vi "subMFD_Design & Analysis.vi"() -> ()   [LabVIEW 2023]
uses:
  <vilib>/Utility/error.llb/ErrWarn.ctl
  <vilib>/addons/Digital Filter Design/_Objects.llb/DFD Filter Ripple Specification (Design).ctl
  <vilib>/addons/Digital Filter Design/_Objects.llb/DFD Multirate Filter Obj.ctl
  <vilib>/addons/Digital Filter Design/_Objects.llb/DFD Multirate Mode.ctl
  <vilib>/addons/Digital Filter Design/_Objects.llb/DFD Coef Norm Type.ctl
  <vilib>/addons/Digital Filter Design/_Objects.llb/DFD Round-off Mode.ctl
  <vilib>/addons/Digital Filter Design/_Objects.llb/DFD FXP MRate Multiply Mode.ctl
  <vilib>/addons/Digital Filter Design/_Objects.llb/DFD Multirate Filter Specification (Design).ctl
  <vilib>/addons/Digital Filter Design/_Objects.llb/DFD Phase Setting.ctl
  <vilib>/addons/Digital Filter Design/Design.llb/DFD MRate Filter Design (Integer).vi
  <vilib>/addons/Digital Filter Design/Design.llb/DFD MRate Filter Design (Rational).vi
  <vilib>/addons/Digital Filter Design/FilterLib.llb/DFD Load MRate Filter from File.vi
  <vilib>/addons/Digital Filter Design/NI_DigFilterLicensed.lvlib
panel:
  out "Status":string="Click the Design button to apply the new specifications."
  out "error":T1=TRUE
  in  "Unwrap?":bool=TRUE
  out "Filter Order":i32=-1
  in  "Magnitude in dB?":bool=TRUE
  in  "Graph Selector":u16(ring) items=["Magnitude", "Phase", "Impulse Response"]
  out "Graph Tab":enum32{"Magnitude", "Phase", "Coefficients"}(tab)
  out "Magnitude Response":cluster{"f0":dbl, "df":dbl, "values":dbl[]}[](graph)
  out "Phase Response":cluster{"f0":dbl, "df":dbl, "values":dbl[]}[](graph)
  out "Coefficients":dbl[](graph)
  out "multirate filter out":T2={"mMRate_Structure"=enum."FIR", "mMRate_Mode"=0, "mMRate_Factor"=-1, "mMRate_FIRParams"={"mMRate_FIR_H"=[], "mMRate_FIR_IsNyquist?"=FALSE, "mMRate_FIR_IsSymmetric?"=FALSE}, "mMRate_CICParams"={"mMRate_CIC_#Stage"=0, "mMRate_CIC_Lag"=1, "mMRate_CIC_Type"=enum."Lowpass"}, "mMRate_Order"=0, "mMRate_Version"="2.0", "mMRate_Comments"="", "mMRate_RationalFactor"={"mMRate_L"=-1, "mMRate_M"=-1}, "mMRate_Fs"=1.0, "mMRate_Quantized?"=FALSE, "mMRate_QFilterGain"=1.0, "mMRate_CoefWl"=16, "mMRate_Scaling"={"mMRate_ScaleByPowerOf2?"=FALSE, "mMRate_ScaleType"=enum."No Norm"}, "mMRate_InputWl"=16, "mMRate_OutputWl"=16, "mMRate_OutputMode"=enum."Truncation", "mMRate_MultMode"=enum."Truncated", "mMRate_BitPruning"=FALSE, "mMRate_GainWl"=16, "mMRate_OutputFwl"=0, "mMRate_SumIwl"=0, "mMRate_InputIwl "=16, "mMRate_SumWl"=32, "mMRate_CoefIwl"=0} {"mMRate_SumWl" min=1 max=32 step=1; "mMRate_InputIwl" min=1 max=32 step=1; "mMRate_GainWl" min=1 max=32 step=1; "mMRate_OutputWl" min=1 max=32 step=1; "mMRate_InputWl" min=1 max=32 step=1; "mMRate_CoefWl" min=1 max=32 step=1; "mMRate_Mode" items=["Default"=-1, "No Rate Change"=0, "Interpolation"=1, "Decimation"=2, "Interpolated"=3, "Rational"=4]}
  in  "freq specs [Hz]":T7={"fpass"=45.0, "fstop"=52.0}
  in  "Get a filter":T8(tab)
  out "fs  out":dbl=48000.0 format="%#_5p Hz"
  in  "fstop":dbl=5000.0 format="%#_5p Hz"
  in  "fs in":dbl=48000.0 format="%#_5p Hz"
  in  "fpass":dbl=4000.0 format="%#_5p Hz"
  in  "Stopband Attenuation":dbl=80.0 format="%#_5g"
  in  "Passband ripple":dbl=0.1 format="%#_5g"
  in  "Design Method":u16(ring) items=["Kaiser Window", "Dolph-Chebyshev Window", "Equi-Ripple FIR"]
  in  "Ripple Specifications in dB?":bool=TRUE
  in  "L 1":i32=1 caption="L" min=1 step=1
  in  "M 1":i32=3 caption="M" min=1 step=1
  out "Flow Diagram 1":u16(ring)=2
  in  "Filter Type 1":u16(ring)=2 items=["No Rate Change", "Interpolation", "Decimation", "Rational resampling"]
  in  "Design":bool
  out "Coefficients Report":string
  out "Filter Type 2":u16(ring)=2 items=["No Rate Change", "Interpolation", "Decimation", "Rational resampling"]
  out "Flow Diagram 2":u16(ring)=2
  out "L 2":i32=1 caption="L" min=1 step=1
  out "M 2":i32=3 caption="M" min=1 step=1
  in  "Load Multirate Filter from File":bool
  in  "multirate filter in":T2={"mMRate_Structure"=enum."FIR", "mMRate_Mode"=0, "mMRate_Factor"=-1, "mMRate_FIRParams"={"mMRate_FIR_H"=[], "mMRate_FIR_IsNyquist?"=FALSE, "mMRate_FIR_IsSymmetric?"=FALSE}, "mMRate_CICParams"={"mMRate_CIC_#Stage"=0, "mMRate_CIC_Lag"=1, "mMRate_CIC_Type"=enum."Lowpass"}, "mMRate_Order"=0, "mMRate_Version"="2.0", "mMRate_Comments"="", "mMRate_RationalFactor"={"mMRate_L"=-1, "mMRate_M"=-1}, "mMRate_Fs"=1.0, "mMRate_Quantized?"=FALSE, "mMRate_QFilterGain"=1.0, "mMRate_CoefWl"=16, "mMRate_Scaling"={"mMRate_ScaleByPowerOf2?"=FALSE, "mMRate_ScaleType"=enum."No Norm"}, "mMRate_InputWl"=16, "mMRate_OutputWl"=16, "mMRate_OutputMode"=enum."Truncation", "mMRate_MultMode"=enum."Truncated", "mMRate_BitPruning"=FALSE, "mMRate_GainWl"=16, "mMRate_OutputFwl"=0, "mMRate_SumIwl"=0, "mMRate_InputIwl "=16, "mMRate_SumWl"=32, "mMRate_CoefIwl"=0} {"mMRate_SumWl" min=1 max=32 step=1; "mMRate_InputIwl" min=1 max=32 step=1; "mMRate_GainWl" min=1 max=32 step=1; "mMRate_OutputWl" min=1 max=32 step=1; "mMRate_InputWl" min=1 max=32 step=1; "mMRate_CoefWl" min=1 max=32 step=1; "mMRate_Mode" items=["Default"=-1, "No Rate Change"=0, "Interpolation"=1, "Decimation"=2, "Interpolated"=3, "Rational"=4]}
  in  "ripple specs":T9={"passband"=0.0, "stopband"=0.0, "dB/linear? (T: dB)"=TRUE}
  out "Successful Design?":bool
  in  "stop":bool
  out "OK":bool
  # "Design Result"
  # "Status"
  # "Filter Specifications"
  # "Filter Type"
  # "Frequency Specifications"
  # "Ripple Specifications"
  # "Design Method"
  # "fs out"
  # "fstop"
  # "fs in"
  # "fpass"
  # "Stopband\nAttenuation"
  # "Passband\nRipple"
  # "Design Result"
  # "Status"
  # "Filter Information"
  # "Filter Type"
  # "Filter Coefficients Report"
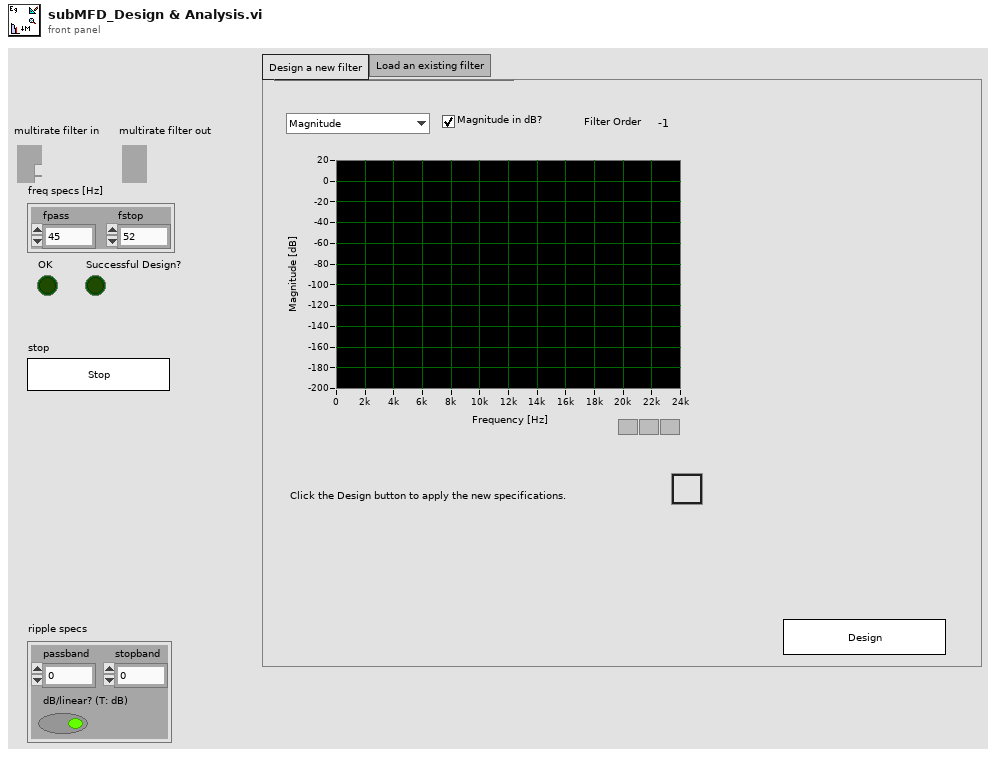
[diagram p1: front panel]
types:
  T1 = typedef "ErrWarn.ctl" = bool
  T2 = typedef "NI_DigFilterLicensed.lvlib/DFD Multirate Filter Obj.ctl" = cluster{"mMRate_Structure":enum16{"CIC", "FIR", "IIR", "Lattice"}, "mMRate_Mode":T3, "mMRate_Factor":i32, "mMRate_FIRParams":cluster{"mMRate_FIR_H":dbl[], "mMRate_FIR_IsNyquist?":bool, "mMRate_FIR_IsSymmetric?":bool}, "mMRate_CICParams":cluster{"mMRate_CIC_#Stage":i32, "mMRate_CIC_Lag":i32, "mMRate_CIC_Type":enum16{"Lowpass", "Highpass"}}, "mMRate_Order":i32, "mMRate_Version":string, "mMRate_Comments":string, "mMRate_RationalFactor":cluster{"mMRate_L":i32, "mMRate_M":i32}, "mMRate_Fs":dbl, "mMRate_Quantized?":bool, "mMRate_QFilterGain":dbl, "mMRate_CoefWl":i16, "mMRate_Scaling":cluster{"mMRate_ScaleByPowerOf2?":bool, "mMRate_ScaleType":T4}, "mMRate_InputWl":i16, "mMRate_OutputWl":i16, "mMRate_OutputMode":T5, "mMRate_MultMode":T6, "mMRate_BitPruning":bool, "mMRate_GainWl":i16, "mMRate_OutputFwl":i16, "mMRate_SumIwl":i16, "mMRate_InputIwl ":i16, "mMRate_SumWl":i16, "mMRate_CoefIwl":i16}
  T3 = typedef "NI_DigFilterLicensed.lvlib/DFD Multirate Mode.ctl" = i16
  T4 = typedef "NI_DigFilterLicensed.lvlib/DFD Coef Norm Type.ctl" = enum16{"No Norm", "Time Domain 1-Norm", "Time Domain 2-Norm", "Time Domain Inf-Norm"}
  T5 = typedef "NI_DigFilterLicensed.lvlib/DFD Round-off Mode.ctl" = enum16{"Nearest", "Truncation"}
  T6 = typedef "NI_DigFilterLicensed.lvlib/DFD FXP MRate Multiply Mode.ctl" = enum16{"Truncated", "Full"}
  T7 = typedef "NI_DigFilterLicensed.lvlib/DFD Multirate Filter Specification (Design).ctl" = cluster{"fpass":dbl, "fstop":dbl}
  T8 = enum32{"Design a new filter", "Load an existing filter"}
  T9 = typedef "NI_DigFilterLicensed.lvlib/DFD Filter Ripple Specification (Design).ctl" = cluster{"passband":dbl, "stopband":dbl, "dB/linear? (T: dB)":bool}
  T10 = typedef "NI_DigFilterLicensed.lvlib/DFD Phase Setting.ctl" = cluster{"unwrap? (F)":bool, "degree? (F)":bool}
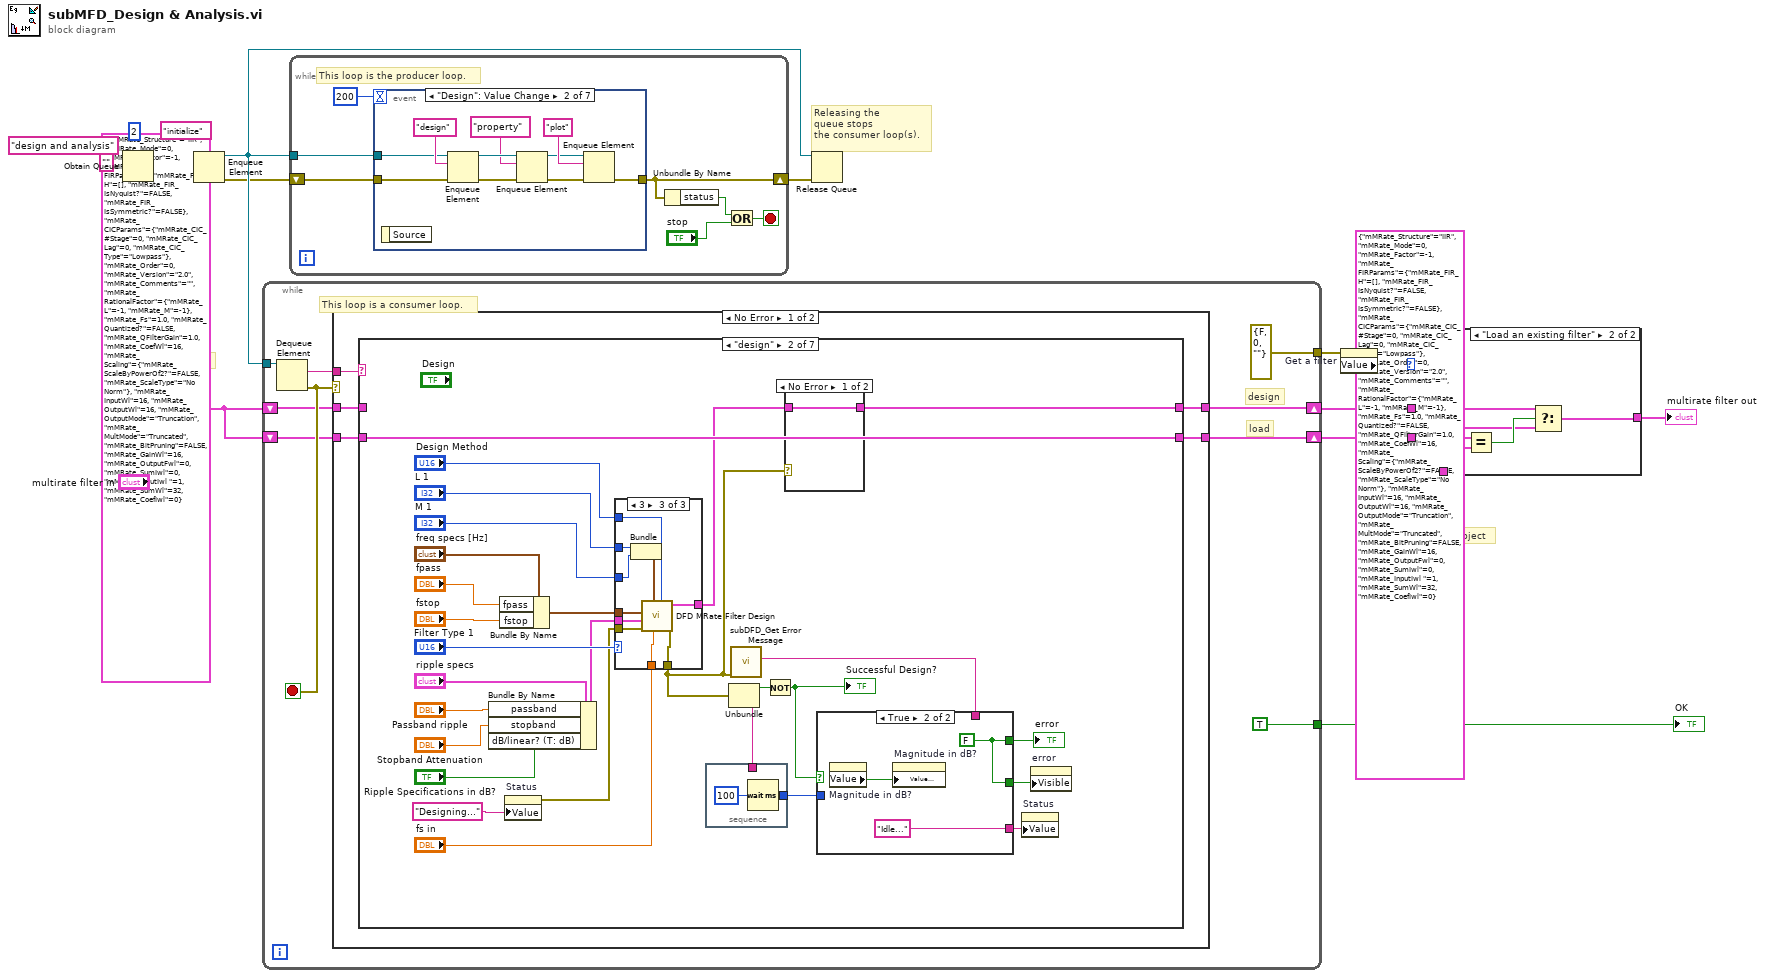
[diagram p0: block diagram]
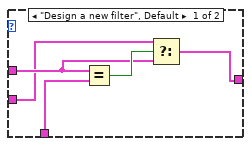
[diagram p2: hidden frame]
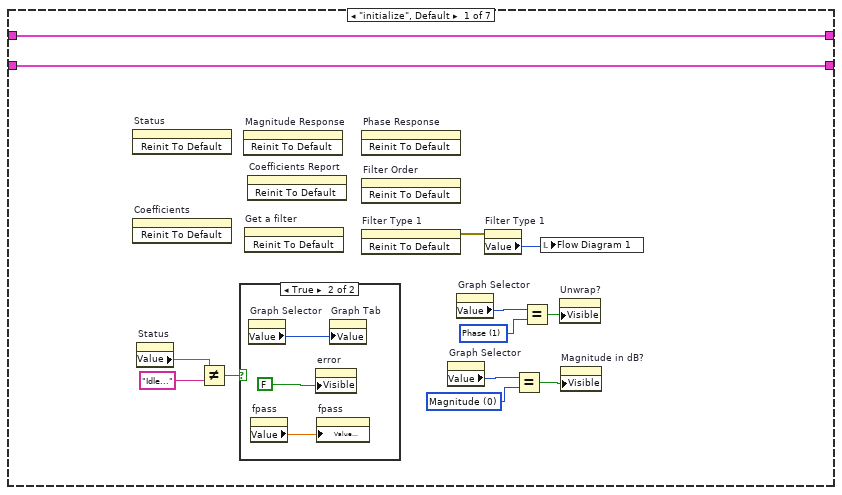
[diagram p3: hidden frame]
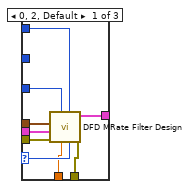
[diagram p6: hidden frame]
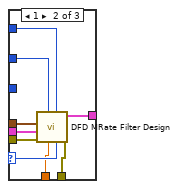
[diagram p7: hidden frame]
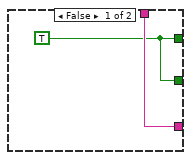
[diagram p8: hidden frame]
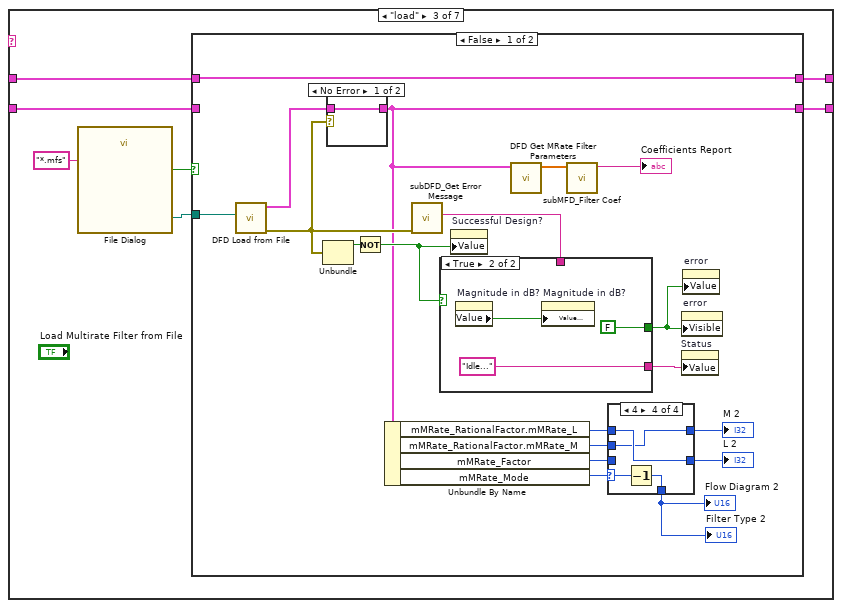
[diagram p9: hidden frame]
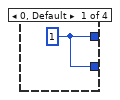
[diagram p10: hidden frame]
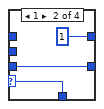
[diagram p11: hidden frame]
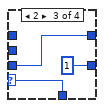
[diagram p12: hidden frame]
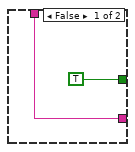
[diagram p14: hidden frame]
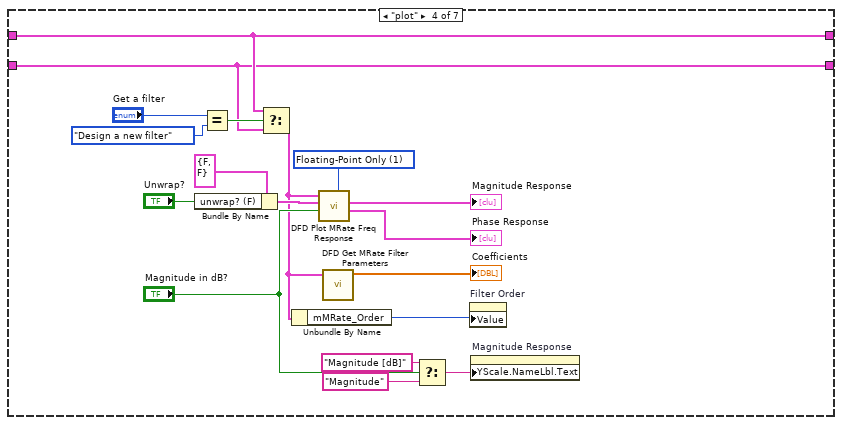
[diagram p16: hidden frame]
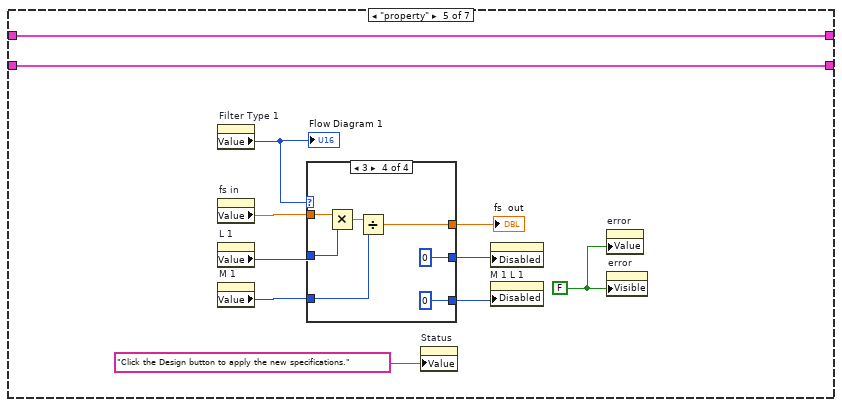
[diagram p17: hidden frame]
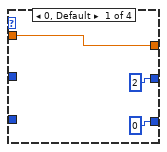
[diagram p18: hidden frame]
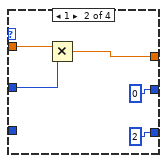
[diagram p19: hidden frame]
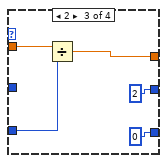
[diagram p20: hidden frame]
diagram:
  w7 = T2 {"mMRate_Structure"=enum."IIR", "mMRate_Mode"=0, "mMRate_Factor"=-1, "mMRate_FIRParams"={"mMRate_FIR_H"=[], "mMRate_FIR_IsNyquist?"=FALSE, "mMRate_FIR_IsSymmetric?"=FALSE}, "mMRate_CICParams"={"mMRate_CIC_#Stage"=0, "mMRate_CIC_Lag"=0, "mMRate_CIC_Type"=enum."Lowpass"}, "mMRate_Order"=0, "mMRate_Version"="2.0", "mMRate_Comments"="", "mMRate_RationalFactor"={"mMRate_L"=-1, "mMRate_M"=-1}, "mMRate_Fs"=1.0, "mMRate_Quantized?"=FALSE, "mMRate_QFilterGain"=1.0, "mMRate_CoefWl"=16, "mMRate_Scaling"={"mMRate_ScaleByPowerOf2?"=FALSE, "mMRate_ScaleType"=enum."No Norm"}, "mMRate_InputWl"=16, "mMRate_OutputWl"=16, "mMRate_OutputMode"=enum."Truncation", "mMRate_MultMode"=enum."Truncated", "mMRate_BitPruning"=FALSE, "mMRate_GainWl"=16, "mMRate_OutputFwl"=0, "mMRate_SumIwl"=0, "mMRate_InputIwl "=1, "mMRate_SumWl"=32, "mMRate_CoefIwl"=0} ("multirate filter out")
  # "empty filter object"
  # "empty filter object"
  # "Releasing the\nqueue stops\nthe consumer loop(s)."
  n1 = Obtain Queue(max queue size (-1, unlimited)=2, name (unnamed)="design and analysis", element data type="" ("name (unnamed)")) -> (queue out=w13:refnum<queue>, error out=w14:errorcluster)  [unwired: 2 in, 1 out]
  n2 = Enqueue Element(queue=w13, element="initialize", error in (no error)=w14) -> (queue out=w12:refnum<queue>, error out=w11:errorcluster)  [unwired: 2 out]
  n3 = while {
    tunnel: w12 -> [w26]
    shift-right: [w23] -> w4
    shift-left: w7 -> [w22]
    tunnel: [TRUE] -> w9
    shift-right: [w19] -> w3
    shift-left: w7 -> [w20]
    tunnel: [errorcluster {"status"=FALSE, "code"=0, "source"=""} ("error in (no error)")] -> w6
    stop <- w25 stop-if-true
    # "load"
    # "design"
    # "This loop is a consumer loop."
    n4 = Dequeue Element(queue=w26) -> (element=w24:string, error out=w25:errorcluster)  [unwired: 1 in, 3 out]
    n5 = case shown="No Error" w25 {
      tunnel: w24 -> [w31 _]
      tunnel: [w30 w229] -> w23
      tunnel: w22 -> [w29 w229]
      tunnel: w20 -> [w28 w228]
      tunnel: [w27 w228] -> w19
      frame No Error {
        n6 = case shown="\"design\"" w31 {
          tunnel: [w41 w50 w114 w160 w185 w210 w222] -> w30
          tunnel: w29 -> [w41 _ w115 w160 w185 w210 w222]
          tunnel: w28 -> [w34 w52 w113 w159 w177 w206 w221]
          tunnel: [w34 w52 w112 w159 w177 w206 w221] -> w27
          frame "initialize", Default {
            w35 = u16 1 items=["Magnitude", "Phase", "Group Delay", "Pole-Zero Plot", "Impulse Response"] ("Graph Selector")
            w39 = u16 0 items=["Magnitude", "Phase", "Group Delay", "Pole-Zero Plot", "Impulse Response"] ("Graph Selector")
            n7 = invoke on="Status" class="Str" method="Reinit To Default"() -> ()  [unwired: 3 in, 3 out]
            n8 = invoke on="Coefficients" class="WFGraph (strict)" method="Reinit To Default"() -> ()  [unwired: 3 in, 3 out]
            n9 = property on="Status" class="Str"() -> ("Value"=w42:string)  [unwired: 2 in, 2 out]
            n10 = Not Equal?(x=w42, y="Idle...") -> (x != y?=w44:bool)
            n11 = case shown="True" w44 {
              frame False {
              }
              frame True {
                n12 = property on="Graph Selector" class="Ring (strict)"() -> ("Value"=w46:u16)  [unwired: 2 in, 2 out]
                n13 = property on="fpass" class="DigNum (strict)"() -> ("Value"=w47:dbl)  [unwired: 2 in, 2 out]
                n14 = property on="error" class="Bool"("Visible"=FALSE) -> ()  [unwired: 2 in, 2 out]
                n15 = property on="fpass" class="DigNum (strict)"("Value (Signaling)"=w47) -> ()  [unwired: 2 in, 2 out]
                n16 = property on="Graph Tab" class="TabCtl (strict)"("Value"=w46) -> ()  [unwired: 2 in, 2 out]
              }
            }
            n17 = invoke on="Magnitude Response" class="WFGraph (strict)" method="Reinit To Default"() -> ()  [unwired: 3 in, 3 out]
            n18 = invoke on="Get a filter" class="TabCtl (strict)" method="Reinit To Default"() -> ()  [unwired: 3 in, 3 out]
            n19 = invoke on="Coefficients Report" class="Str" method="Reinit To Default"() -> ()  [unwired: 3 in, 3 out]
            n20 = invoke on="Phase Response" class="WFGraph (strict)" method="Reinit To Default"() -> ()  [unwired: 3 in, 3 out]
            n21 = invoke on="Filter Order" class="DigNum (strict)" method="Reinit To Default"() -> ()  [unwired: 3 in, 3 out]
            n22 = invoke on="Filter Type 1" class="Ring (strict)" method="Reinit To Default"() -> (error out=w33:errorcluster)  [unwired: 3 in, 2 out]
            n23 = property on="Graph Selector" class="Ring (strict)"() -> ("Value"=w40:u16)  [unwired: 2 in, 2 out]
            n24 = property on="Graph Selector" class="Ring (strict)"() -> ("Value"=w36:u16)  [unwired: 2 in, 2 out]
            n25 = property on="Filter Type 1" class="Ring (strict)"(error in=w33) -> ("Value"=w32:u16)  [unwired: 1 in, 2 out]
            n26 = Equal?(x=w40, y=w39) -> (x = y?=w38:bool)
            n27 = Equal?(x=w36, y=w35) -> (x = y?=w37:bool)
            n28 = local write "Flow Diagram 1"(w32) -> ()
            n29 = property on="Unwrap?" class="Bool (strict)"("Visible"=w37) -> ()  [unwired: 2 in, 2 out]
            n30 = property on="Magnitude in dB?" class="Bool (strict)"("Visible"=w38) -> ()  [unwired: 2 in, 2 out]
          }
          frame "design" {
            n31 = Bundle By Name(cluster="ripple specs", "passband"="Passband ripple", "stopband"="Stopband Attenuation", "dB/linear? (T: dB)"="Ripple Specifications in dB?") -> (w56:T9)
            n32 = Bundle By Name(cluster="freq specs [Hz]", "fpass"="fpass", "fstop"="fstop") -> (w58:T7)
            n33 = property on="Status" class="Str"("Value"="Designing..." ("status")) -> (error out=w55:errorcluster)  [unwired: 2 in, 1 out]
            n34 = case shown="3" "Filter Type 1" {
              selector: "Filter Type 1" -> [w80 w89 _]
              tunnel: w58 -> [w85 w94 w95]
              tunnel: w56 -> [w84 w93 w104]
              tunnel: "fs in" -> [w78 w87 w103]
              tunnel: w55 -> [w83 w92 w102]
              tunnel: [w82 w91 w101] -> w51
              tunnel: "Design Method" -> [w81 w90 w100]
              tunnel: [w79 w88 w99] -> w53
              tunnel: "L 1" -> [_ w86 w97]
              tunnel: "M 1" -> [w77 _ w98]
              frame 0, 2, Default {
                n35 = call-poly <vilib>:"DFD MRate Filter Design.vi"("filtering mode"=w80, "method"=w81, "fs in [Hz]"=w78, "factor"=w77, "error in (no error)"=w83, "ripple specs"=w84, "freq specs [Hz]"=w85) -> ("error out"=w79:errorcluster, "multirate filter out"=w82:T2)  [unwired: 1 in, 2 out]
              }
              frame 1 {
                n36 = call-poly <vilib>:"DFD MRate Filter Design.vi"("filtering mode"=w89, "method"=w90, "fs in [Hz]"=w87, "factor"=w86, "error in (no error)"=w92, "ripple specs"=w93, "freq specs [Hz]"=w94) -> ("error out"=w88:errorcluster, "multirate filter out"=w91:T2)  [unwired: 1 in, 2 out]
              }
              frame 3 {
                n37 = Bundle("L 1"=w97, "M 1"=w98) -> (w96:cluster{"L 1":i32, "M 1":i32})  [unwired: 1 out]
                n38 = call-poly <vilib>:"DFD MRate Filter Design.vi"("method"=w100, "fs in [Hz]"=w103, "factor"=w96, "error in (no error)"=w102, "ripple specs"=w104, "freq specs [Hz]"=w95) -> ("error out"=w99:errorcluster, "multirate filter out"=w101:T2)  [unwired: 1 in, 3 out]
              }
            }
            n39 = Unbundle(w53) -> ("status"=w67:bool, "source"=w71:string)  [unwired: 1 out]
            n40 = stacked-sequence {
              tunnel: w71 -> [_]
              tunnel: [w105] -> w72
              frame #0 {
                n41 = Wait (ms)(milliseconds to wait=u32 100) -> (millisecond timer value=w105:u32)
              }
            }
            n42 = call <vilib>:"subDFD_Get Error Message.vi"("error in (no error)"=w53) -> ("Error Message"=w75:string)  [unwired: 10 out]
            n43 = Not(x=w67) -> (.not. x?=w68:bool)
            "Successful Design?" <- w68
            n44 = case shown="No Error" w53 {
              tunnel: w51 -> [w76 _]
              tunnel: [w76 _] -> w50
              frame No Error {
              }
              frame Error {
              }
            }
            n45 = case shown="True" w68 {
              tunnel: [w108 "Idle..." ("status")] -> w70
              tunnel: w72 -> [_ _]
              tunnel: w75 -> [w108 _]
              tunnel: [w107 w109] -> w49
              tunnel: [w107 w109] -> w48
              frame False {
                w107 = T1 TRUE ("error")
              }
              frame True {
                w109 = T1 FALSE ("error")
                n46 = property on="Magnitude in dB?" class="Bool (strict)"() -> ("Value"=w111:bool)  [unwired: 2 in, 2 out]
                n47 = property on="Magnitude in dB?" class="Bool (strict)"("Value (Signaling)"=w111) -> ()  [unwired: 2 in, 2 out]
              }
            }
            "error" <- w49
            n48 = property on="Status" class="Str"("Value"=w70) -> ()  [unwired: 2 in, 2 out]
            n49 = property on="error" class="Bool"("Visible"=w48) -> ()  [unwired: 2 in, 2 out]
          }
          frame "load" {
            n50 = call "File Dialog"("pattern (all files)"="*.mfs") -> ("selected path"=w118:path, "cancelled"=w117:bool)  [unwired: 6 in, 7 out]
            n51 = case shown="False" w117 {
              tunnel: w115 -> [w122 w156]
              tunnel: [w122 w156] -> w114
              tunnel: w118 -> [w132 _]
              tunnel: w113 -> [_ w155]
              tunnel: [w121 w155] -> w112
              frame False {
                n52 = call-poly <vilib>:"DFD Load from File.vi"("file path in"=w132) -> ("error out"=w130:errorcluster, "multirate filter out"=w123:T2)  [unwired: 1 in, 8 out]
                n53 = Unbundle(w130) -> ("status"=w137:bool)  [unwired: 2 out]
                n54 = case shown="No Error" w130 {
                  tunnel: w123 -> [w149 _]
                  tunnel: [w149 _] -> w121
                  frame No Error {
                  }
                  frame Error {
                  }
                }
                n55 = Not(x=w137) -> (.not. x?=w136:bool)
                n56 = Unbundle By Name(w121) -> ("mMRate_RationalFactor.mMRate_L"=w129:i32, "mMRate_RationalFactor.mMRate_M"=w128:i32, "mMRate_Factor"=w127:i32, "mMRate_Mode"=w124:T3)
                n57 = call <vilib>:"subDFD_Get Error Message.vi"("error in (no error)"=w130) -> ("Error Message"=w135:string)  [unwired: 10 out]
                n58 = case shown="True" w136 {
                  tunnel: [w151 "Idle..." ("status")] -> w131
                  tunnel: w135 -> [w151 _]
                  tunnel: [TRUE ("Visible") FALSE ("Visible")] -> w120
                  frame False {
                  }
                  frame True {
                    n59 = property on="Magnitude in dB?" class="Bool (strict)"() -> ("Value"=w154:bool)  [unwired: 2 in, 2 out]
                    n60 = property on="Magnitude in dB?" class="Bool (strict)"("Value (Signaling)"=w154) -> ()  [unwired: 2 in, 2 out]
                  }
                }
                n61 = property on="Successful Design?" class="Bool (strict)"("Value"=w136) -> ()  [unwired: 2 in, 2 out]
                n62 = call <vilib>:"DFD Get MRate Filter Parameters.vi"("multirate filter in"=w121) -> ("h(n)"=w133:dbl[])  [unwired: 2 in, 8 out]
                n63 = call "subMFD_Filter Coef.vi"("h(n)"=w133) -> ("Coefficients Report"=→"Coefficients Report":string)  [unwired: 1 in, 9 out]
                n64 = case shown="4" w124 {
                  selector: w124 -> [_ w139 w142 w146]
                  tunnel: w129 -> [_ _ _ w148]
                  tunnel: w128 -> [_ _ _ w147]
                  tunnel: w127 -> [_ w140 w143 _]
                  tunnel: [w138 1 ("M 2") w143 w147] -> w126
                  tunnel: [w138 w140 1 ("mMRate_Factor") w148] -> w125
                  tunnel: [_ w139 w142 w145] -> w119
                  frame 0, Default {
                    w138 = 1 ("mMRate_M")
                  }
                  frame 1 {
                  }
                  frame 2 {
                  }
                  frame 4 {
                    n65 = Decrement(x=w146) -> (x-1=w145:T3)
                  }
                }
                "M 2" <- w126
                "L 2" <- w125
                "Flow Diagram 2" <- w119
                "Filter Type 2" <- w119
                n66 = property on="error" class="Bool"("Visible"=w120) -> ()  [unwired: 2 in, 2 out]
                n67 = property on="Status" class="Str"("Value"=w131) -> ()  [unwired: 2 in, 2 out]
                n68 = property on="error" class="Bool"("Value"=w120) -> ()  [unwired: 2 in, 2 out]
              }
              frame True {
              }
            }
          }
          frame "plot" {
            w167 = u16 1 items=["Auto", "Floating-Point Only", "Fixed-Point Only"] ("output option")
            n69 = Bundle By Name(cluster=T10 {"unwrap? (F)"=FALSE, "degree? (F)"=FALSE} ("phase view"), "unwrap? (F)"="Unwrap?") -> (w168:T10)
            n70 = Equal?(x="Get a filter", y=T8."Design a new filter") -> (x = y?=w161:bool)
            n71 = Select(t=w160, s=w161, f=w159) -> (s? t:f=w158:T2)
            n72 = Unbundle By Name(w158) -> ("mMRate_Order"=w157:i32)
            n73 = call <vilib>:"DFD Plot MRate Freq Response.vi"("output option"=w167, "dB on? (T)"="Magnitude in dB?", "phase view"=w168, "multirate filter in"=w158) -> ("phase response"=→"Phase Response":cluster{"f0":dbl, "df":dbl, "values":dbl[]}[], "magnitude response"=→"Magnitude Response":cluster{"f0":dbl, "df":dbl, "values":dbl[]}[])  [unwired: 3 in, 3 out]
            n74 = call <vilib>:"DFD Get MRate Filter Parameters.vi"("multirate filter in"=w158) -> ("h(n)"=→"Coefficients":dbl[])  [unwired: 2 in, 8 out]
            n75 = Select(t="Magnitude [dB]", s="Magnitude in dB?", f="Magnitude") -> (s? t:f=w174:string)
            n76 = property on="Filter Order" class="DigNum (strict)"("Value"=w157) -> ()  [unwired: 2 in, 2 out]
            n77 = property on="Magnitude Response" class="WFGraph (strict)"("YScale.NameLbl.Text"=w174) -> ()  [unwired: 2 in, 2 out]
          }
          frame "property" {
            w176 = FALSE ("Visible")
            n78 = property on="Filter Type 1" class="Ring (strict)"() -> ("Value"=w178:u16)  [unwired: 2 in, 2 out]
            "Flow Diagram 1" <- w178
            n79 = property on="fs in" class="DigNum (strict)"() -> ("Value"=w184:dbl)  [unwired: 2 in, 2 out]
            n80 = property on="L 1" class="DigNum (strict)"() -> ("Value"=w183:i32)  [unwired: 2 in, 2 out]
            n81 = property on="M 1" class="DigNum (strict)"() -> ("Value"=w182:i32)  [unwired: 2 in, 2 out]
            n82 = case shown="3" w178 {
              tunnel: w184 -> [w188 w193 w198 w203]
              tunnel: w183 -> [_ w192 _ w202]
              tunnel: w182 -> [_ _ w196 w204]
              tunnel: [w188 w191 w197 w205] -> w179
              tunnel: [u8 2 ("Disabled") u8 0 ("Disabled") u8 2 ("Disabled") u8 0 ("Disabled")] -> w181
              tunnel: [u8 0 ("Disabled") u8 2 ("Disabled") u8 0 ("Disabled") u8 0 ("Disabled")] -> w180
              frame 0, Default {
              }
              frame 1 {
                n83 = Multiply(x=w193, y=w192) -> (x*y=w191:dbl)
              }
              frame 2 {
                n84 = Divide(x=w198, y=w196) -> (x/y=w197:dbl)
              }
              frame 3 {
                n85 = Multiply(x=w203, y=w202) -> (x*y=w201:dbl)
                n86 = Divide(x=w201, y=w204) -> (x/y=w205:dbl)
              }
            }
            "fs  out" <- w179
            n87 = property on="Status" class="Str"("Value"="Click the Design button to apply the new specifications.") -> ()  [unwired: 2 in, 2 out]
            n88 = property on="L 1" class="DigNum (strict)"("Disabled"=w181) -> ()  [unwired: 2 in, 2 out]
            n89 = property on="M 1" class="DigNum (strict)"("Disabled"=w180) -> ()  [unwired: 2 in, 2 out]
            n90 = property on="error" class="Bool"("Value"=w176) -> ()  [unwired: 2 in, 2 out]
            n91 = property on="error" class="Bool"("Visible"=w176) -> ()  [unwired: 2 in, 2 out]
          }
          frame "graph selector" {
            n92 = case shown="1" "Graph Selector" {
              tunnel: [FALSE TRUE FALSE] -> w208
              tunnel: [TRUE FALSE FALSE] -> w207
              frame 0 {
              }
              frame 1 {
              }
              frame 2, Default {
              }
            }
            n93 = property on="Unwrap?" class="Bool (strict)"("Visible"=w208) -> ()  [unwired: 2 in, 2 out]
            n94 = property on="Magnitude in dB?" class="Bool (strict)"("Visible"=w207) -> ()  [unwired: 2 in, 2 out]
            "Graph Tab" <- "Graph Selector"
          }
          frame "switch method" {
            w217 = FALSE ("Visible")
            n95 = property on="Get a filter" class="TabCtl (strict)"() -> ("Value"=w227:T8)  [unwired: 2 in, 2 out]
            n96 = Equal?(x=w227, y=T8."Design a new filter") -> (x = y?=w220:bool)
            n97 = Select(t="Click the Design button to apply the new specifications.", s=w220, f="Click the Load Multirate Filter from File button to load an existing filter.") -> (s? t:f=→"Status":string)
            n98 = Select(t=w222, s=w220, f=w221) -> (s? t:f=w219:T2)
            n99 = Unbundle By Name(w219) -> ("mMRate_Order"=→"Filter Order":i32)
            n100 = property on="error" class="Bool"("Value"=w217) -> ()  [unwired: 2 in, 2 out]
            n101 = property on="error" class="Bool"("Visible"=w217) -> ()  [unwired: 2 in, 2 out]
          }
        }
      }
      frame Error {
      }
    }
  }
  "OK" <- w9
  n102 = while {
    shift-right: [w233] -> w17
    shift-left: w11 -> [w235]
    tunnel: w12 -> [w236]
    stop <- w234 stop-if-true
    # "This loop is the producer loop."
    n103 = event shown="[1] \"Design\": Value Change" {
      selector: _ -> [_ _ _ _ _ _ _]
      dyn-events: _ -> [_ _ _ _ _ _ _]
      timeout: 200 -> [_ _ _ _ _ _ _]
      tunnel: w236 -> [w242 w252 w254 w261 w265 w271 _]
      tunnel: w235 -> [w241 w251 w257 w260 w264 w270 w273]
      tunnel: [w239 w250 w256 w259 w263 w267 w273] -> w233
      event "Load Multirate Filter from File": Value Change {
        n104 = event-data() -> ()  [unwired: 2 out]
        n105 = Enqueue Element(queue=w242, element="load", error in (no error)=w241) -> (queue out=w238:refnum<queue>, error out=w240:errorcluster)  [unwired: 2 out]
        n106 = Enqueue Element(queue=w238, element="plot", error in (no error)=w240) -> (error out=w239:errorcluster)  [unwired: 3 out]
      }
      event "Design": Value Change {
        n107 = event-data() -> ()  [unwired: 2 out]
        n108 = Enqueue Element(queue=w252, element="design", error in (no error)=w251) -> (queue out=w248:refnum<queue>, error out=w246:errorcluster)  [unwired: 2 out]
        n109 = Enqueue Element(queue=w248, element="property", error in (no error)=w246) -> (queue out=w247:refnum<queue>, error out=w245:errorcluster)  [unwired: 2 out]
        n110 = Enqueue Element(queue=w247, element="plot", error in (no error)=w245) -> (error out=w250:errorcluster)  [unwired: 3 out]
      }
      event "Magnitude in dB?", "Unwrap?": Value Change {
        n111 = event-data() -> ()  [unwired: 2 out]
        n112 = Enqueue Element(queue=w254, element="plot", error in (no error)=w257) -> (error out=w256:errorcluster)  [unwired: 3 out]
      }
      event "Graph Selector": Value Change {
        n113 = event-data() -> ()  [unwired: 2 out]
        n114 = Enqueue Element(queue=w261, element="graph selector", error in (no error)=w260) -> (error out=w259:errorcluster)  [unwired: 3 out]
      }
      event "fs in", "L 1", "M 1", "Filter Type 1": Value Change {
        n115 = event-data() -> ()  [unwired: 2 out]
        n116 = Enqueue Element(queue=w265, element="property", error in (no error)=w264) -> (error out=w263:errorcluster)  [unwired: 3 out]
      }
      event "Get a filter": Value Change {
        n117 = event-data() -> ()  [unwired: 2 out]
        n118 = Enqueue Element(queue=w271, element="switch method", error in (no error)=w270) -> (queue out=w266:refnum<queue>, error out=w268:errorcluster)  [unwired: 2 out]
        n119 = Enqueue Element(queue=w266, element="plot", error in (no error)=w268) -> (error out=w267:errorcluster)  [unwired: 3 out]
      }
      event Timeout {
        n120 = event-data() -> ()  [unwired: 2 out]
      }
    }
    n121 = Unbundle By Name(w233) -> ("status"=w232:bool)
    n122 = Or(x=w232, y="stop") -> (x .or. y?=w234:bool)
  }
  n123 = Release Queue(queue=w12, error in (no error)=w17) -> ()  [unwired: 4 out]
  n124 = property on="Get a filter" class="TabCtl (strict)"(error in=w6) -> ("Value"=w5:T8)  [unwired: 1 in, 2 out]
  n125 = case shown="\"Load an existing filter\"" w5 {
    tunnel: w4 -> [w276 w281]
    tunnel: w3 -> [w275 w280]
    tunnel: T2 {"mMRate_Structure"=enum."IIR", "mMRate_Mode"=0, "mMRate_Factor"=-1, "mMRate_FIRParams"={"mMRate_FIR_H"=[], "mMRate_FIR_IsNyquist?"=FALSE, "mMRate_FIR_IsSymmetric?"=FALSE}, "mMRate_CICParams"={"mMRate_CIC_#Stage"=0, "mMRate_CIC_Lag"=0, "mMRate_CIC_Type"=enum."Lowpass"}, "mMRate_Order"=0, "mMRate_Version"="2.0", "mMRate_Comments"="", "mMRate_RationalFactor"={"mMRate_L"=-1, "mMRate_M"=-1}, "mMRate_Fs"=1.0, "mMRate_Quantized?"=FALSE, "mMRate_QFilterGain"=1.0, "mMRate_CoefWl"=16, "mMRate_Scaling"={"mMRate_ScaleByPowerOf2?"=FALSE, "mMRate_ScaleType"=enum."No Norm"}, "mMRate_InputWl"=16, "mMRate_OutputWl"=16, "mMRate_OutputMode"=enum."Truncation", "mMRate_MultMode"=enum."Truncated", "mMRate_BitPruning"=FALSE, "mMRate_GainWl"=16, "mMRate_OutputFwl"=0, "mMRate_SumIwl"=0, "mMRate_InputIwl "=1, "mMRate_SumWl"=32, "mMRate_CoefIwl"=0} ("multirate filter out") -> [w277 w283]
    tunnel: [w274 w279] -> w1
    frame "Design a new filter", Default {
      n126 = Equal?(x=w276, y=w277) -> (x = y?=w278:bool)
      n127 = Select(t=w275, s=w278, f=w276) -> (s? t:f=w274:T2)
    }
    frame "Load an existing filter" {
      n128 = Equal?(x=w280, y=w283) -> (x = y?=w282:bool)
      n129 = Select(t=w281, s=w282, f=w280) -> (s? t:f=w279:T2)
    }
  }
  "multirate filter out" <- w1
